vi "Find First Tag Header.vi"(8 "Error In":errorcluster, 11 "XML String":string) -> (0 "Error Out":errorcluster, 3 "After First Tag String":string, 4 "Parsing Info":T2, 5 "Parsed Header":T1)   [LabVIEW 2017, in "Tree API.lvlib" / "Tree.lvclass"]
uses:
  Tree.lvclass
  Parsing Info.ctl
  <vilib>/ErrorRing/Error Ring.xnode
  Parsed Header.ctl
  <vilib>/Utility/error.llb/Error Cluster From Error Code.vi
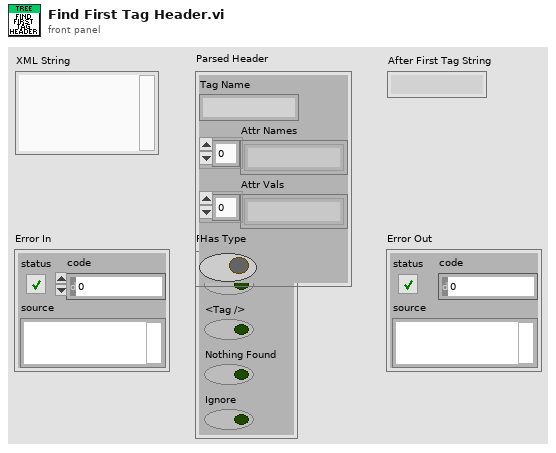
[diagram p1: front panel]
types:
  T1 = typedef "Tree API.lvlib/Tree.lvclass/Parsed Header.ctl" = cluster{"Tag Name":string, "Attr Names":string[], "Attr Vals":string[], "Has Type":bool}
  T2 = typedef "Tree API.lvlib/Tree.lvclass/Parsing Info.ctl" = cluster{"</ Tag>":bool, "<Tag />":bool, "Nothing Found":bool, "Ignore":bool}
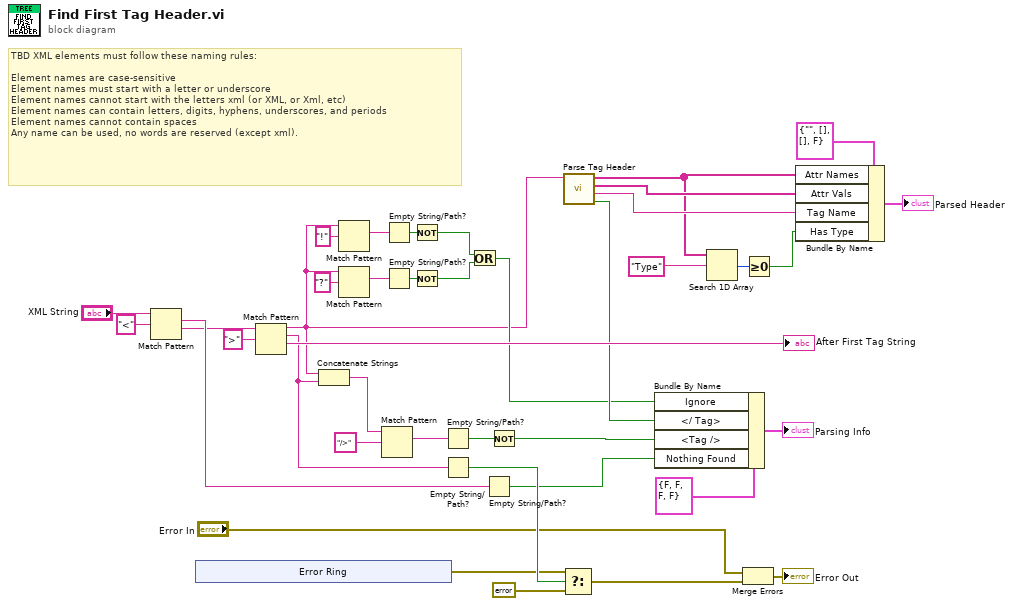
[diagram p0: block diagram]
diagram:
  # "TBD XML elements must follow these naming rules:\n\nElement names are case-sensitive\nElement names must start with a letter or underscore\nElement names cannot start with the letters xml (or XML, or Xml, etc)\nElement names can contain letters, digits, hyphens, underscores, and periods\nElement names cannot contain spaces\nAny name can be used, no words are reserved (except xml)."
  n1 = Match Pattern(string="XML String", regular expression="<") -> (match substring=w37:string, after substring=w10:string)  [unwired: 1 in, 2 out]
  n2 = xnode "Error Ring"() -> ("错误输出"=w26:errorcluster)
  n3 = Match Pattern(string=w10, regular expression=">") -> (before substring=w6:string, match substring=w29:string, after substring=→"After First Tag String":string)  [unwired: 1 in, 1 out]
  n4 = Concatenate Strings(w6, w29) -> (w28:string)
  n5 = Match Pattern(string=w6, regular expression="!") -> (match substring=w12:string)  [unwired: 1 in, 3 out]
  n6 = Match Pattern(string=w6, regular expression="?") -> (match substring=w15:string)  [unwired: 1 in, 3 out]
  n7 = Match Pattern(string=w28, regular expression="/>") -> (match substring=w35:string)  [unwired: 1 in, 3 out]
  n8 = Empty String/Path?(string/path=w12) -> (empty?=w13:bool)
  n9 = Empty String/Path?(string/path=w15) -> (empty?=w14:bool)
  n10 = Not(x=w13) -> (.not. x?=w8:bool)
  n11 = Not(x=w14) -> (.not. x?=w9:bool)
  n12 = Empty String/Path?(string/path=w35) -> (empty?=w32:bool)
  n13 = Empty String/Path?(string/path=w29) -> (empty?=w27:bool)
  n14 = Or(x=w8, y=w9) -> (x .or. y?=w7:bool)
  n15 = Empty String/Path?(string/path=w37) -> (empty?=w24:bool)
  n16 = Not(x=w32) -> (.not. x?=w25:bool)
  n17 = Select(t=w26, s=w27, f=errorcluster {"status"=FALSE, "code"=0, "source"=""}) -> (s? t:f=w20:errorcluster)
  n18 = call "Parse Tag Header.vi"("Tag Header String"=w6) -> ("</ Tag>"=w33:bool, "Tag Name"=w5:string, "Attr Vals"=w22:string[], "Attr Names"=w3:string[])  [unwired: 7 in]
  n19 = Bundle By Name(cluster=T2 {"</ Tag>"=FALSE, "<Tag />"=FALSE, "Nothing Found"=FALSE, "Ignore"=FALSE}, "Ignore"=w7, "</ Tag>"=w33, "<Tag />"=w25, "Nothing Found"=w24) -> (→"Parsing Info":T2)
  n20 = Search 1D Array(1D array=w3, element="Type") -> (index of element=w2:i32)  [unwired: 1 in]
  n21 = Merge Errors("Error In", w20) -> (→"Error Out":errorcluster)
  n22 = Greater Or Equal To 0?(x=w2) -> (x >= 0?=w1:bool)
  n23 = Bundle By Name(cluster=T1 {"Tag Name"="", "Attr Names"=[], "Attr Vals"=[], "Has Type"=FALSE} ("output cluster"), "Attr Names"=w3, "Attr Vals"=w22, "Tag Name"=w5, "Has Type"=w1) -> (→"Parsed Header":T1)
